vi "Close Handle.vi"(8 "error in":errorcluster, 11 "Win32 Event in":refnum<class "Win32 Event.lvclass">) -> (0 "error out":errorcluster, 3 "Win32 Event out":refnum<class "Win32 Event.lvclass">)   [LabVIEW 2019, in "PCANBasic.lvlib" / "Win32 Event.lvclass"]
doc: "If the function succeeds, the return value is a handle to the event object."
uses:
  Win32 Event.lvclass
  Win32 Event.lvclass/Win32 Event.ctl
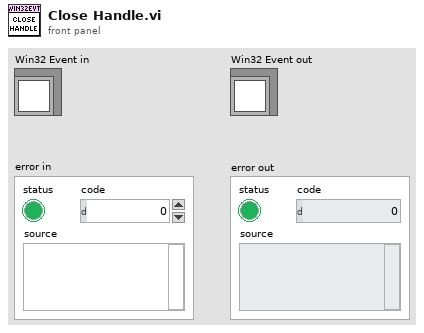
[diagram p1: front panel]
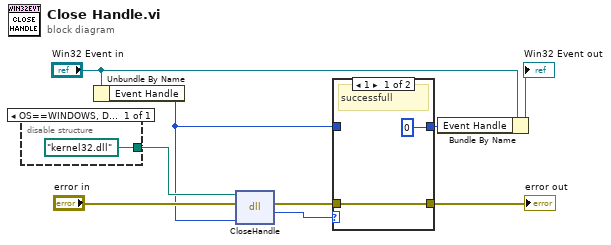
[diagram p0: block diagram]
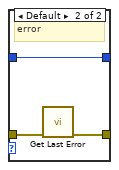
[diagram p2: hidden frame]
diagram:
  n1 = disable-structure shown="OS==WINDOWS, Default" {
    disable-tunnel: [path "kernel32.dll" ("path in")] -> w9
    frame condition #0 (active) {
    }
  }
  n2 = Unbundle By Name("Win32 Event in") -> ("Event Handle"=w1:u64)
  n3 = dll-call lib="?" fn="CloseHandle"(path in=w9, error in="error in", "hdlEvent"=w1) -> (error out=w7:errorcluster, "status"=w5:i32)  [unwired: 2 in, 1 out]
  n4 = case "success?" shown="1" w5 {
    tunnel: w7 -> [w12 w15]
    tunnel: [w12 w14] -> w6
    tunnel: [u64 0 ("Event Handle") w13] -> w2
    tunnel: w1 -> [_ w13]
    frame 1 {
      # "successfull"
    }
    frame Default {
      # "error"
      n5 = call "Get Last Error.vi"("error in"=w15) -> ("error out"=w14:errorcluster)  [unwired: 10 in]
    }
  }
  "error out" <- w6
  n6 = Bundle By Name(cluster="Win32 Event in", "Event Handle"=w2) -> (→"Win32 Event out":refnum<class "Win32 Event.lvclass">)
